vi "画图.vi"   [LabVIEW 2019]
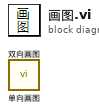
[diagram p0: block diagram]
diagram:
  n1 = call "单向画图.vi"() -> ()  [unwired: 4 in, 1 out]
  n2 = call "双向画图.vi"() -> ()  [unwired: 4 in, 1 out]
